vi "LinesToText.vi"(8 "error in (no error)":errorcluster, 10 "Section(Empty)":string, 11 "Lines":string[](array[string])) -> (0 "error out":errorcluster, 3 "string":string)   [LabVIEW 2012]
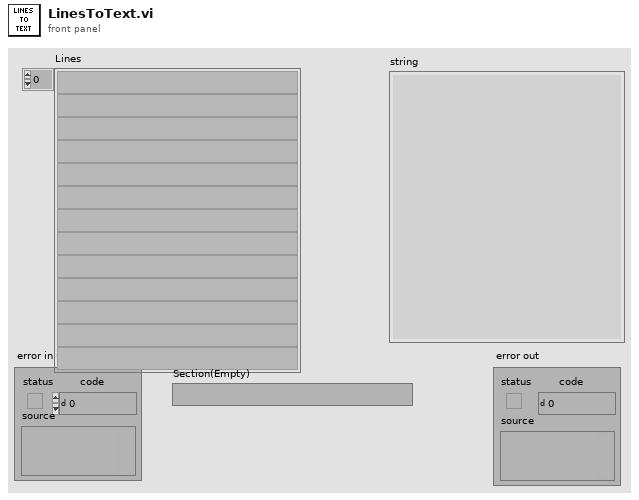
[diagram p1: front panel]
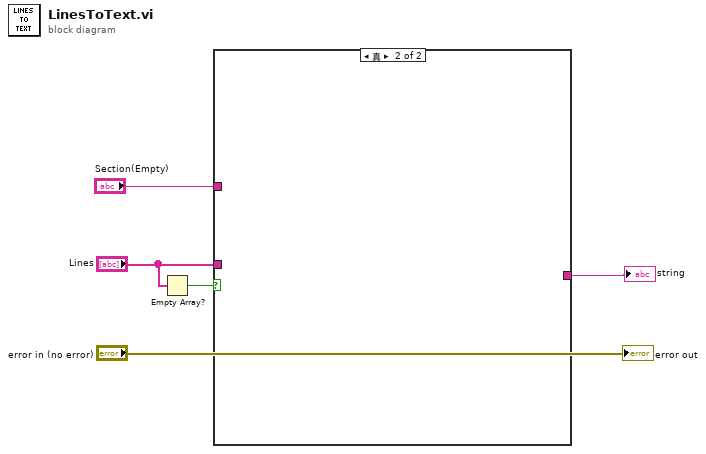
[diagram p0: block diagram]
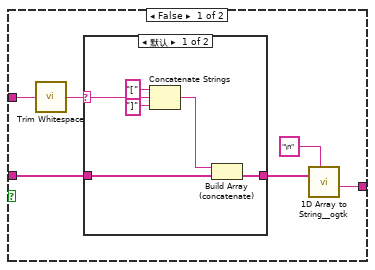
[diagram p2: hidden frame]
diagram:
  n1 = Empty Array?(array="Lines") -> (empty?=w1:bool)
  n2 = case shown="真" w1 {
    tunnel: "Section(Empty)" -> [w10 _]
    tunnel: [w8 _] -> w3
    tunnel: "Lines" -> [w6 _]
    frame False {
      n3 = call <vilib>:"Trim Whitespace.vi"("string"=w10) -> ("trimmed string"=w9:string)  [unwired: 1 in]
      n4 = case shown="默认" w9 {
        selector: w9 -> [w17 _]
        tunnel: [w13 w18] -> w7
        tunnel: w6 -> [w14 w18]
        frame Default {
          n5 = Concatenate Strings("[" ("string"), w17, "]" ("string")) -> (w12:string)
          n6 = Build Array (concatenate)(w12, w14) -> (w13:string[])
        }
        frame "" {
        }
      }
      n7 = call <userlib>:"1D Array to String__ogtk.vi"("delimiter (Tab)"="\n", "Array of Strings"=w7) -> ("delimited string"=w8:string)  [unwired: 9 in]
    }
    frame True {
    }
  }
  "string" <- w3
  "error out" <- "error in (no error)"
